vi "DAQ-Events2Case.vi"(2 "DAQ Controls Old":T1={"Minimum Value"=-10.0, "Maximum Value"=10.0, "Physical Channel"="Dev1/ao0", "DAQ Fs (S/s)"=10000.0}, 3 "DAQ Controls New":T1={"Minimum Value"=-10.0, "Maximum Value"=10.0, "Physical Channel"="Dev1/ao0", "DAQ Fs (S/s)"=10000.0}) -> (0 "DAQ Cambio Array":T2(array[ring]), 1 "DAQ Cambio?":bool)   [LabVIEW 2010]
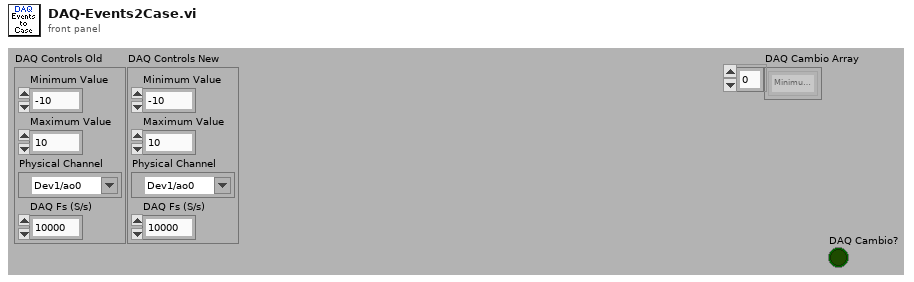
[diagram p1: front panel]
types:
  T1 = cluster{"Minimum Value":dbl, "Maximum Value":dbl, "Physical Channel":tag, "DAQ Fs (S/s)":dbl}
  T2 = enum16{"Minimum Value", "Maximum Value", "Physical Channel", "DAQ Fs", "DAQ ON/OFF", "Nothing"}[]
  T3 = enum16{"Minimum Value", "Maximum Value", "Physical Channel", "DAQ Fs", "DAQ ON/OFF", "Nothing"}
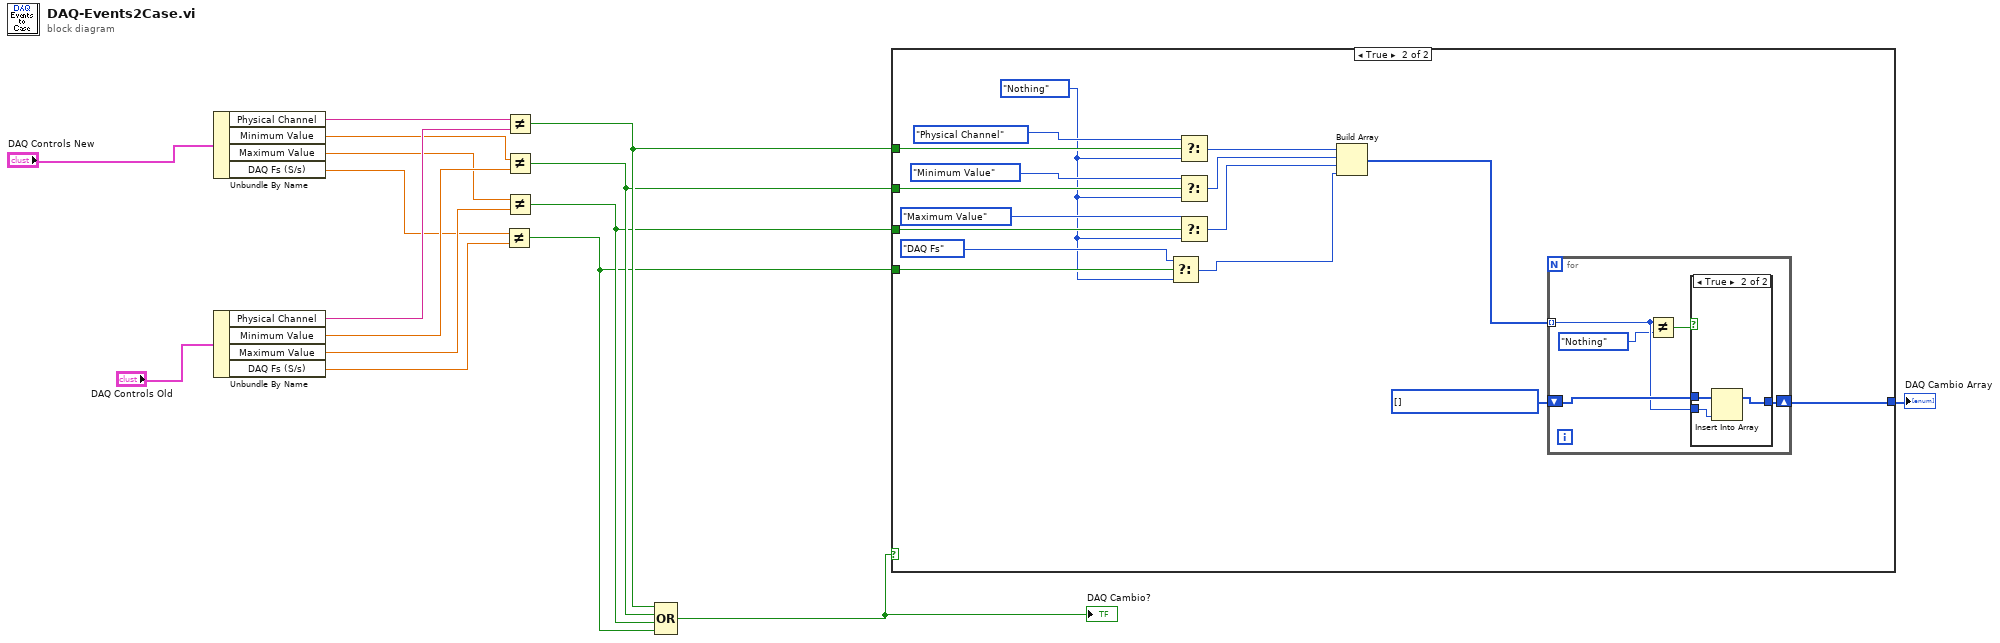
[diagram p0: block diagram]
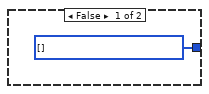
[diagram p2: hidden frame]
diagram:
  n1 = Unbundle By Name("DAQ Controls New") -> ("Physical Channel"=w16:tag, "Minimum Value"=w14:dbl, "Maximum Value"=w12:dbl, "DAQ Fs (S/s)"=w4:dbl)
  n2 = Unbundle By Name("DAQ Controls Old") -> ("Physical Channel"=w15:tag, "Minimum Value"=w13:dbl, "Maximum Value"=w11:dbl, "DAQ Fs (S/s)"=w3:dbl)
  n3 = Not Equal?(x=w4, y=w3) -> (x != y?=w2:bool)
  n4 = Not Equal?(x=w16, y=w15) -> (x != y?=w10:bool)
  n5 = Not Equal?(x=w14, y=w13) -> (x != y?=w9:bool)
  n6 = Not Equal?(x=w12, y=w11) -> (x != y?=w8:bool)
  n7 = Compound Arithmetic op=OR(w10, w9, w8, w2) -> (w7:bool)
  "DAQ Cambio?" <- w7
  n8 = case shown="True" w7 {
    tunnel: w10 -> [_ w30]
    tunnel: w9 -> [_ w27]
    tunnel: w8 -> [_ w29]
    tunnel: [w17 w24] -> w1
    tunnel: w2 -> [_ w25]
    frame False {
      w17 = T2 [] items=["Minimum Value", "Maximum Value", "Physical Channel", "DAQ Fs", "DAQ ON/OFF", "Nothing"]
    }
    frame True {
      w23 = T2 [] items=["Minimum Value", "Maximum Value", "Physical Channel", "DAQ Fs", "DAQ ON/OFF", "Nothing"]
      w18 = T3."Nothing"
      n9 = Select(t=T3."DAQ Fs", s=w25, f=w18) -> (s? t:f=w26:T3)
      n10 = Select(t=T3."Physical Channel", s=w30, f=w18) -> (s? t:f=w33:T3)
      n11 = Select(t=T3."Minimum Value", s=w27, f=w18) -> (s? t:f=w32:T3)
      n12 = Select(t=T3."Maximum Value", s=w29, f=w18) -> (s? t:f=w31:T3)
      n13 = Build Array(w33, w32, w31, w26) -> (w28:T2)
      n14 = for {
        tunnel: w28 -> [w36] mode=indexing
        shift-right: [w35] -> w24
        shift-left: w23 -> [w37]
        n15 = Not Equal?(x=w36, y=T3."Nothing") -> (x != y?=w38:bool)
        n16 = case shown="True" w38 {
          tunnel: w37 -> [w39 w42]
          tunnel: w36 -> [_ w40]
          tunnel: [w39 w41] -> w35
          frame False {
          }
          frame True {
            n17 = Insert Into Array(array=w42, new element=w40) -> (w41:T2)  [unwired: 1 in]
          }
        }
      }
    }
  }
  "DAQ Cambio Array" <- w1
